vi "Status-Background-Thread.vi"(7 "TcpRouter-Client":refnum<class "TcpRouter-Client.lvclass">, 8 "error in (no error)":errorcluster) -> (0 "error out":errorcluster)   [LabVIEW 2020, in "CSM-TCP-Router.lvlib" / "TcpRouter-Client.lvclass"]
uses:
  TcpRouter-Client.lvclass
  TcpRouter-Client.lvclass/TcpRouter-Client.ctl
  Def-TCP-Router Status Data.ctl
  CSM-TCP-Router.lvlib
  <userlib>/_NEVSTOP/Communicable State Machine(CSM)/_Shared/CSM Shared.lvlib
panel:
  out "current time":timestamp
  out "String":string
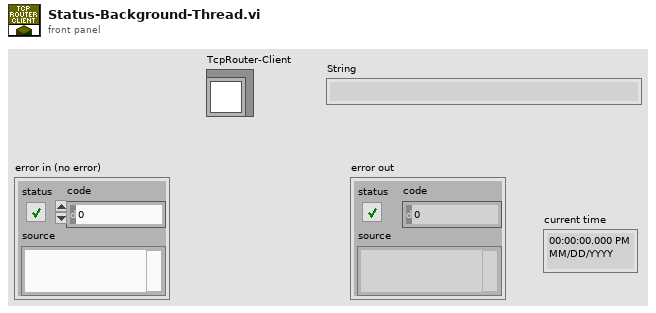
[diagram p1: front panel]
types:
  T1 = typedef "CSM-TCP-Router.lvlib/TcpRouter-Client.lvclass/Def-TCP-Router Status Data.ctl" = cluster{"status":string, "arg":string, "source":string}
  T2 = typedef "CSM-TCP-Router.lvlib/TcpRouter-Client.lvclass/Def-TCP-Router PUB-SUB.ctl" = cluster{"STATUS":refnum<k5>, "StatusQueue":refnum<queue>}
  T3 = typedef "CSM-TCP-Router.lvlib/tcp-msg type.ctl" = enum8{"info", "error", "cmd", "cmd-resp", "resp", "async-resp", "status", "interrupt"}
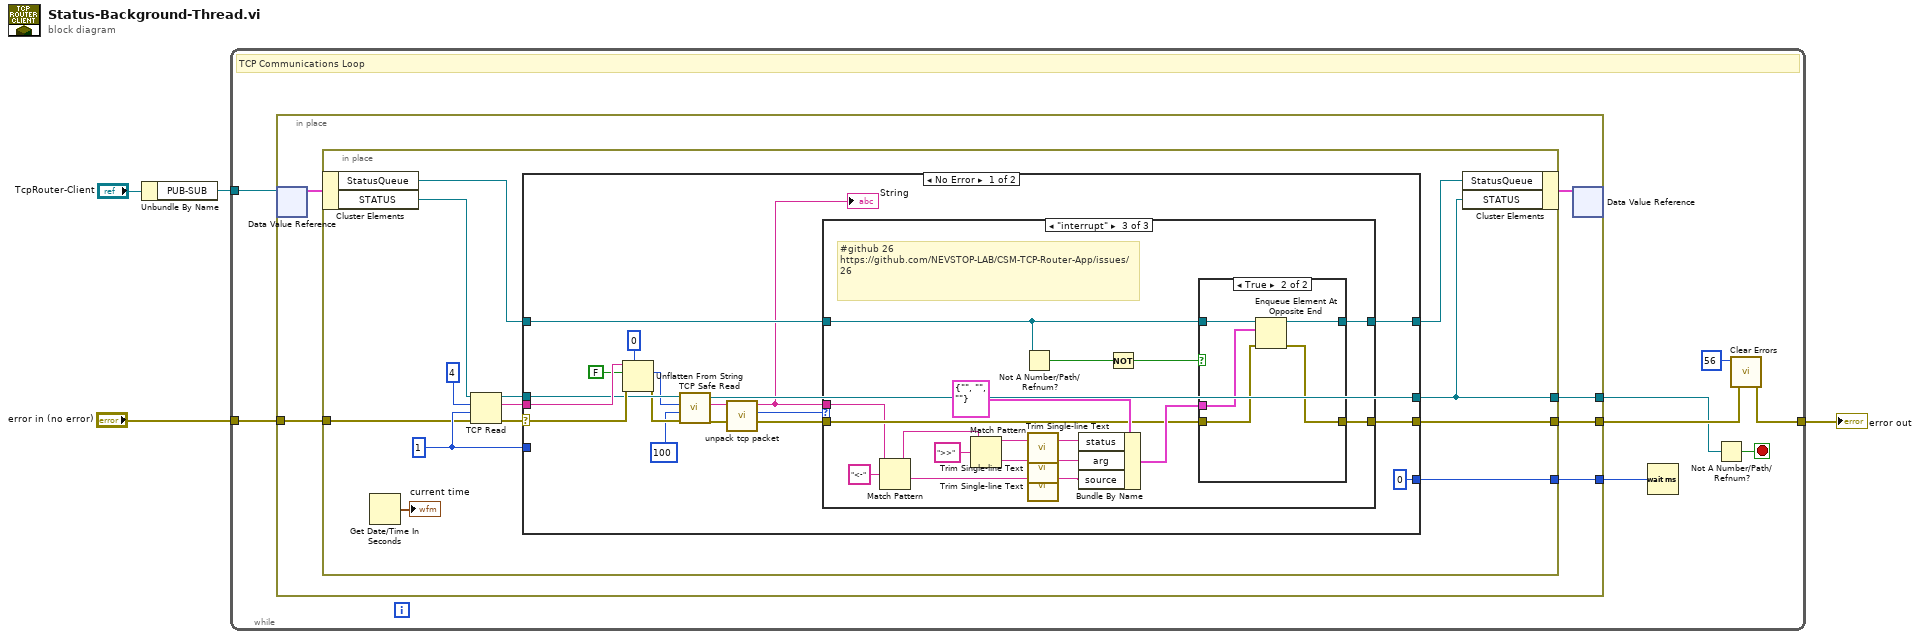
[diagram p0: block diagram]
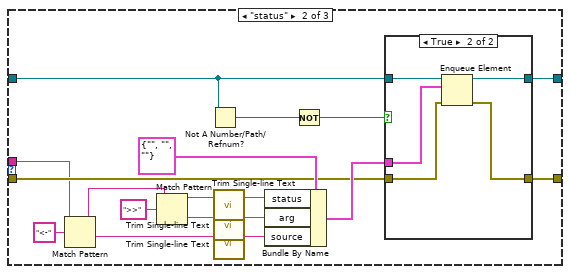
[diagram p3: hidden frame]
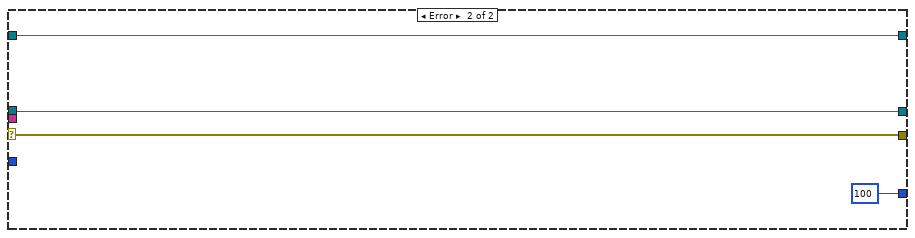
[diagram p6: hidden frame]
diagram:
  n1 = Unbundle By Name("TcpRouter-Client") -> ("PUB-SUB"=w1:refnum<data-value>)
  n2 = while {
    tunnel: [w11] -> w3
    tunnel: "error in (no error)" -> [w8]
    tunnel: w1 -> [w9]
    stop <- w10 stop-if-true
    # "TCP Communications Loop"
    n3 = in-place {
      in-place-border: w8 -> [w16]
      in-place-border: [w15] -> w7
      in-place-border: [w14] -> w6
      in-place-border: [w13] -> w5
      n4 = in-place-dvr #1(w9) -> (w18:T2)  [unwired: 1 out]
      n5 = in-place {
        in-place-border: w16 -> [w23]
        in-place-border: [w22] -> w15
        in-place-border: [w21] -> w14
        in-place-border: [w20] -> w13
        w27 = 1 ("timeout ms (1000)")
        n6 = in-place-cluster #2(w18) -> ("StatusQueue"=w26:refnum<queue>, "STATUS"=w24:refnum<k5>)
        n7 = Get Date/Time In Seconds() -> (seconds since 1Jan1904=→"current time":timestamp)
        n8 = TCP Read(connection ID=w24, bytes to read=4, error in (no error)=w23, 9:w27) -> (connection ID out=w29:refnum<k5>, data out=w30:string, error out=w31:errorcluster)  [unwired: 1 in]
        n9 = case shown="No Error" w31 {
          selector: w31 -> [w46 w104]
          tunnel: [w48 w103] -> w21
          tunnel: [w36 w104] -> w22
          tunnel: [w47 w102] -> w25
          tunnel: w30 -> [w45 _]
          tunnel: w29 -> [w44 w103]
          tunnel: w27 -> [_ _]
          tunnel: w26 -> [w35 w102]
          tunnel: [u32 0 ("milliseconds to wait") u32 100 ("milliseconds to wait")] -> w20
          frame No Error {
            n10 = Unflatten From String(type=0, binary string=w45, data includes array or string size? (T)=FALSE, error in (no error)=w46) -> (value=w42:i32, error out=w41:errorcluster)  [unwired: 2 out]
            n11 = call "TCP Safe Read.vi"("error in (no error)"=w41, "timeout ms (25000)"=100 ("timeout ms (1000)"), "bytes to read"=w42, "TCP Network Connection in"=w44) -> ("error out"=w37:errorcluster, "String"=w43:string, "TCP Network Connection out"=w48:refnum<k5>)  [unwired: 5 in]
            n12 = call "unpack tcp packet.vi"("TCP Pack"=w43) -> ("tcp-message-type"=w38:T3, "String"=w32:string)  [unwired: 9 in]
            "String" <- w32
            n13 = case shown="\"interrupt\"" w38 {
              tunnel: [w49 w68 w93] -> w47
              tunnel: w32 -> [_ w61 w86]
              tunnel: w37 -> [w50 w65 w90]
              tunnel: [w50 w64 w89] -> w36
              tunnel: w35 -> [w49 w63 w88]
              frame Default {
              }
              frame "status" {
                n14 = Match Pattern(string=w61, regular expression="<-") -> (before substring=w57:string, after substring=w59:string)  [unwired: 1 in, 2 out]
                n15 = Match Pattern(string=w57, regular expression=">>") -> (before substring=w56:string, after substring=w55:string)  [unwired: 1 in, 2 out]
                n16 = Not A Number/Path/Refnum?(number/path/refnum=w63) -> (NaN/Path/Refnum?=w62:bool)
                n17 = call <userlib>:"Trim Single-line Text.vi"("single-line text"=w56) -> ("trimed text"=w52:string)  [unwired: 2 in]
                n18 = call <userlib>:"Trim Single-line Text.vi"("single-line text"=w55) -> ("trimed text"=w53:string)  [unwired: 2 in]
                n19 = call <userlib>:"Trim Single-line Text.vi"("single-line text"=w59) -> ("trimed text"=w58:string)  [unwired: 2 in]
                n20 = Bundle By Name(cluster=T1 {"status"="", "arg"="", "source"=""} ("Cluster"), "status"=w52, "arg"=w53, "source"=w58) -> (w66:T1)
                n21 = Not(x=w62) -> (.not. x?=w51:bool)
                n22 = case shown="True" w51 {
                  tunnel: [w70 w75] -> w68
                  tunnel: w66 -> [_ w74]
                  tunnel: w65 -> [w69 w73]
                  tunnel: [w69 w72] -> w64
                  tunnel: w63 -> [w70 w71]
                  frame False {
                  }
                  frame True {
                    n23 = Enqueue Element(queue=w71, element=w74, error in (no error)=w73) -> (queue out=w75:refnum<queue>, error out=w72:errorcluster)  [unwired: 1 in, 1 out]
                  }
                }
              }
              frame "interrupt" {
                # "#github 26\nhttps://github.com/NEVSTOP-LAB/CSM-TCP-Router-App/issues/26"
                n24 = Match Pattern(string=w86, regular expression="<-") -> (before substring=w82:string, after substring=w84:string)  [unwired: 1 in, 2 out]
                n25 = Match Pattern(string=w82, regular expression=">>") -> (before substring=w81:string, after substring=w80:string)  [unwired: 1 in, 2 out]
                n26 = Not A Number/Path/Refnum?(number/path/refnum=w88) -> (NaN/Path/Refnum?=w87:bool)
                n27 = call <userlib>:"Trim Single-line Text.vi"("single-line text"=w81) -> ("trimed text"=w77:string)  [unwired: 2 in]
                n28 = call <userlib>:"Trim Single-line Text.vi"("single-line text"=w80) -> ("trimed text"=w78:string)  [unwired: 2 in]
                n29 = call <userlib>:"Trim Single-line Text.vi"("single-line text"=w84) -> ("trimed text"=w83:string)  [unwired: 2 in]
                n30 = Bundle By Name(cluster=T1 {"status"="", "arg"="", "source"=""} ("Cluster"), "status"=w77, "arg"=w78, "source"=w83) -> (w91:T1)
                n31 = Not(x=w87) -> (.not. x?=w76:bool)
                n32 = case shown="True" w76 {
                  tunnel: [w95 w100] -> w93
                  tunnel: w91 -> [_ w99]
                  tunnel: w90 -> [w94 w98]
                  tunnel: [w94 w97] -> w89
                  tunnel: w88 -> [w95 w96]
                  frame False {
                  }
                  frame True {
                    n33 = Enqueue Element At Opposite End(queue=w96, element=w99, error in (no error)=w98) -> (queue out=w100:refnum<queue>, error out=w97:errorcluster)  [unwired: 1 in, 1 out]
                  }
                }
              }
            }
          }
          frame Error {
          }
        }
        n34 = in-place-cluster #2("StatusQueue"=w25, "STATUS"=w21) -> (w17:T2)
      }
      n35 = in-place-dvr #1(w17) -> ()  [unwired: 2 out]
    }
    n36 = Wait (ms)(milliseconds to wait=w5) -> ()  [unwired: 1 out]
    n37 = Not A Number/Path/Refnum?(number/path/refnum=w6) -> (NaN/Path/Refnum?=w10:bool)
    n38 = call <vilib>:"Clear Errors.vi"("error in (no error)"=w7, "specific error code to clear (0: all)"=56) -> ("error out"=w11:errorcluster)  [unwired: 4 in, 1 out]
  }
  "error out" <- w3
